vi "AVI Video Save.vi"(5 "Frame Size":u32, 6 "Channel":T1, 7 "AVI mode":T6, 8 "error in (no error)":errorcluster, 9 "AVI cluster":T2, 10 "PMT is ON?":bool, 11 "Image Pixels":i16[][](array[numeric])) -> (0 "error out":errorcluster, 2 "New split file has just been initialised":bool)   [LabVIEW 2017]
uses:
  Typedefs/AVI implementation enum.ctl
  Typedefs/AVI Refs cluster.ctl
  <vilib>/vision/Avi.llb/IMAQ AVI2 Refnum.ctl
  <vilib>/vision/Image Controls.llb/IMAQ Image.ctl
  <vilib>/vision/Avi1.llb/AviRefnum.ctl
  Typedefs/Channel Selector.ctl
  Globals/gl_Binary time series files globals.vi
panel:
  in  "file (use dialog) 2":path=path "X:/Microscope data/2015-July-31/Binary data 2.bin"
  in  "file (use dialog)":path=path "X:/Microscope data/2015-July-31/Binary data 1.bin"
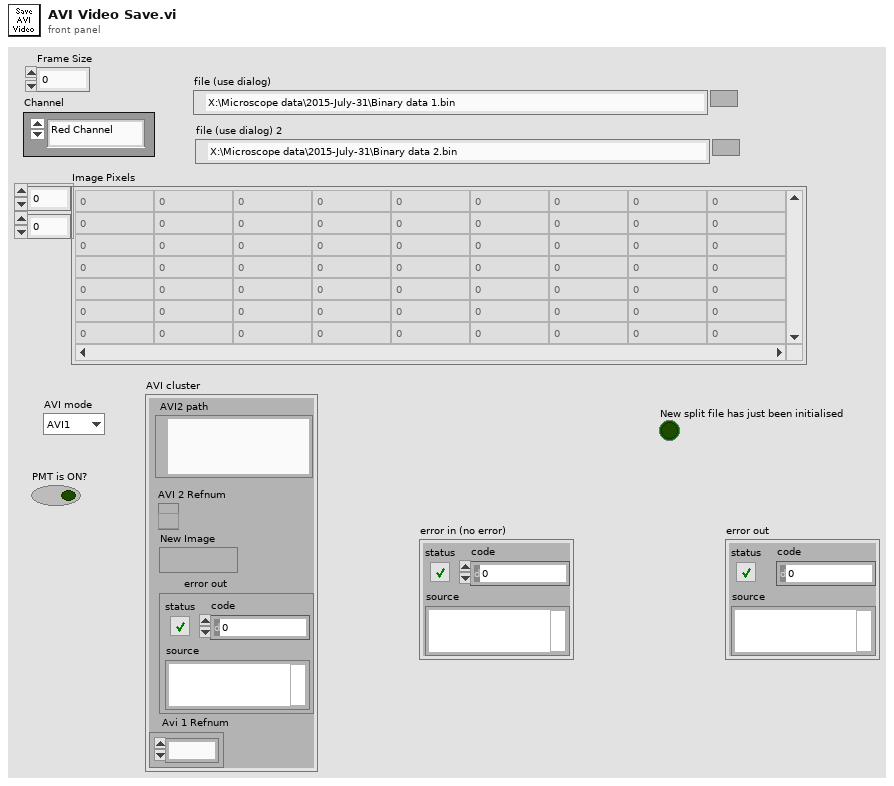
[diagram p1: front panel]
types:
  T1 = typedef "Channel Selector.ctl" = enum16{"Red Channel", "Green Channel", "Blended"}
  T2 = typedef "AVI Refs cluster.ctl" = cluster{"AVI2 path":path, "AVI 2 Refnum":T3, "New Image":T4, "error out":errorcluster, "Avi 1 Refnum":T5}
  T3 = typedef "IMAQ AVI2 Refnum.ctl" = refnum<k20>
  T4 = typedef "IMAQ Image.ctl" = refnum<image>
  T5 = typedef "AviRefnum.ctl" = refnum<k1>
  T6 = typedef "AVI implementation enum.ctl" = enum16{"AVI1", "AVI2"}
  T7 = enum16{"open", "replace", "create", "open or create", "replace or create", "replace or create with confirmation"}
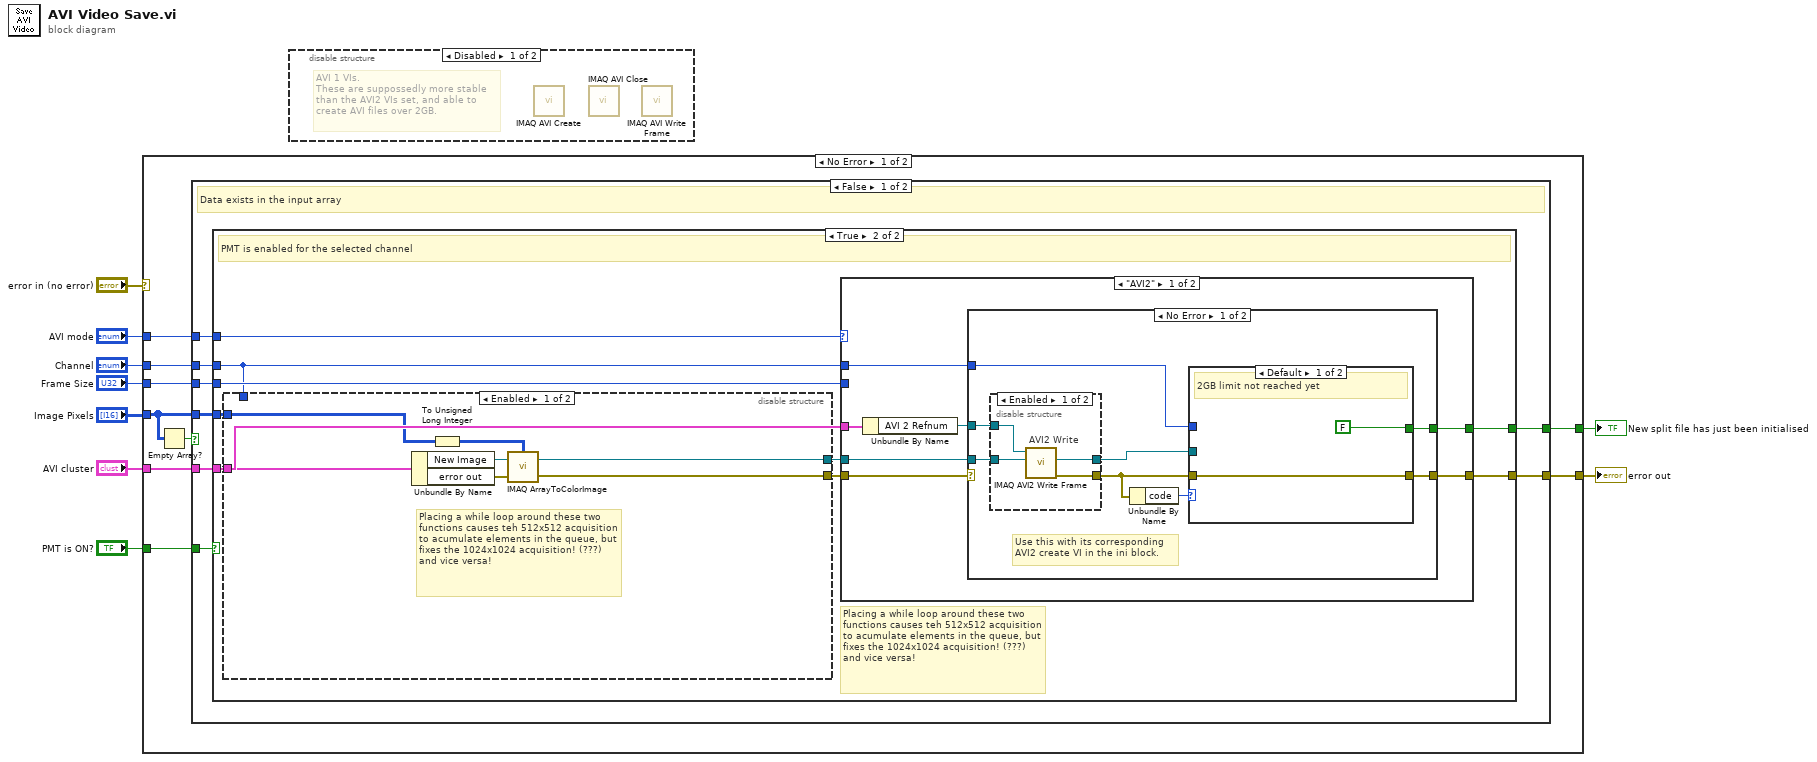
[diagram p0: block diagram]
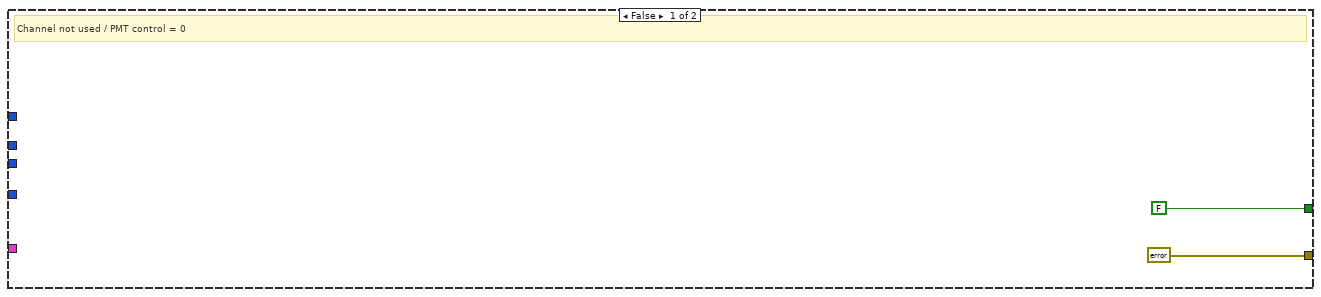
[diagram p3: hidden frame]
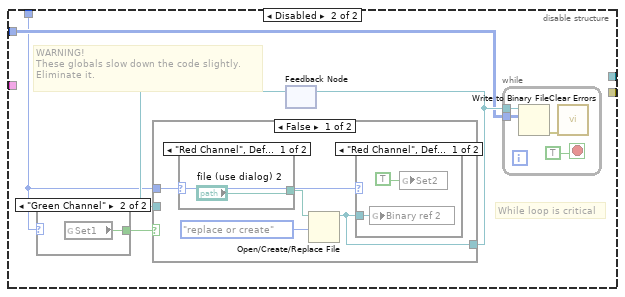
[diagram p4: hidden frame]
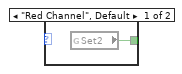
[diagram p5: hidden frame]
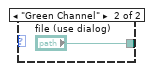
[diagram p6: hidden frame]
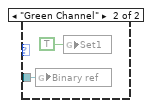
[diagram p7: hidden frame]
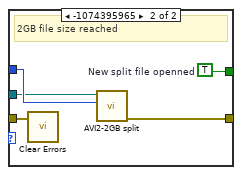
[diagram p10: hidden frame]
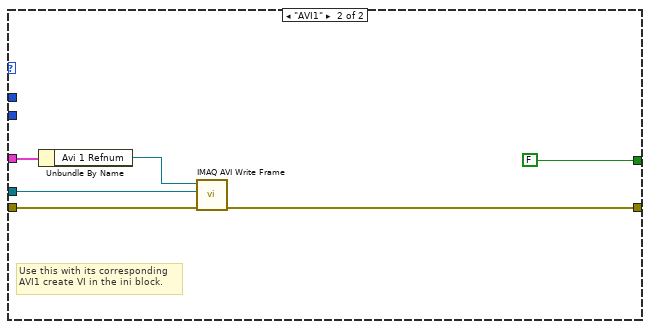
[diagram p12: hidden frame]
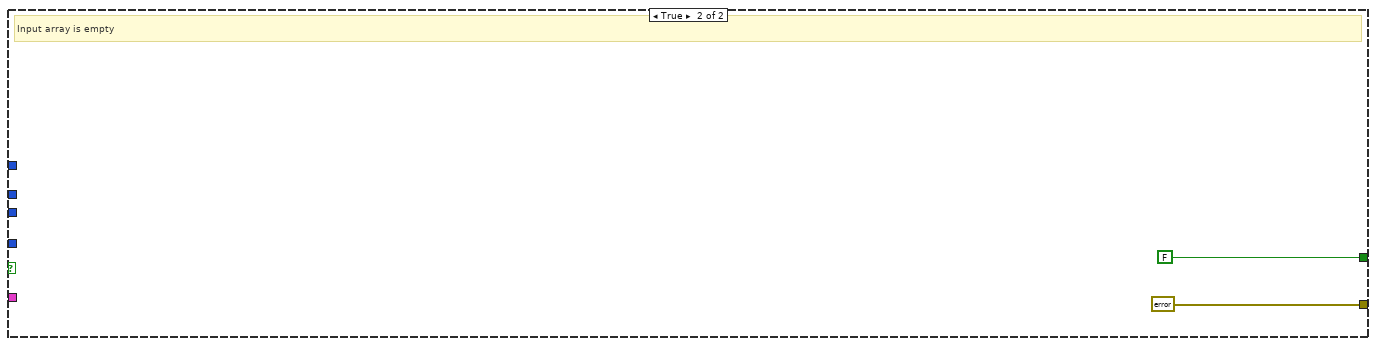
[diagram p13: hidden frame]
diagram:
  n1 = case shown="No Error" "error in (no error)" {
    tunnel: [w18 _] -> w7
    tunnel: "Image Pixels" -> [w10 _]
    tunnel: "AVI mode" -> [w17 _]
    tunnel: "AVI cluster" -> [w16 _]
    tunnel: "PMT is ON?" -> [w15 _]
    tunnel: "Channel" -> [w14 _]
    tunnel: [w13 _] -> w2
    tunnel: "Frame Size" -> [w12 _]
    frame No Error {
      n2 = Empty Array?(array=w10) -> (empty?=w11:bool)
      n3 = case shown="False" w11 {
        tunnel: w10 -> [w26 _]
        tunnel: [w25 errorcluster {"status"=FALSE, "code"=0, "source"=""} ("error out")] -> w18
        tunnel: w17 -> [w24 _]
        tunnel: w16 -> [w23 _]
        tunnel: w15 -> [w22 _]
        tunnel: w14 -> [w21 _]
        tunnel: [w20 FALSE] -> w13
        tunnel: w12 -> [w19 _]
        frame False {
          # "Data exists in the input array"
          n4 = case shown="True" w22 {
            tunnel: w26 -> [_ w30]
            tunnel: w23 -> [_ w33]
            tunnel: [errorcluster {"status"=FALSE, "code"=0, "source"=""} ("error out") w35] -> w25
            tunnel: w24 -> [_ w34]
            tunnel: w21 -> [_ w29]
            tunnel: [FALSE w32] -> w20
            tunnel: w19 -> [_ w31]
            frame False {
              # "Channel not used / PMT control = 0"
            }
            frame True {
              # "Placing a while loop around these two functions causes teh 512x512 acquisition to acumulate elements in the queue, but fixes the 1024x1024 acquisition! (???)  and vice versa!"
              # "PMT is enabled for the selected channel"
              n5 = disable-structure shown="Enabled" {
                disable-tunnel: [w44 _] -> w37
                disable-tunnel: [w43 _] -> w36
                disable-tunnel: w33 -> [w40 _]
                disable-tunnel: w30 -> [w38 w47]
                disable-tunnel: w29 -> [_ w45]
                frame Enabled {
                  # "Placing a while loop around these two functions causes teh 512x512 acquisition to acumulate elements in the queue, but fixes the 1024x1024 acquisition! (???)  and vice versa!"
                  n6 = Unbundle By Name(w40) -> ("New Image"=w42:T4, "error out"=w41:errorcluster)
                  n7 = To Unsigned Long Integer(number=w38) -> (unsigned 32bit integer=w39:u32[][])
                  n8 = call "IMAQ ArrayToColorImage"("Image Pixels (U32)"=w39, "Image"=w42, "error in (no error)"=w41) -> ("Image Out"=w43:T4, "error out"=w44:errorcluster)  [unwired: 1 in, 1 out]
                }
                frame Disabled {
                  # "WARNING!\nThese globals slow down the code slightly.\nEliminate it."
                  # "While loop is critical"
                  n9 = case shown="\"Green Channel\"" w45 {
                    tunnel: [w50 w51] -> w46
                    frame "Red Channel", Default {
                      n10 = global read "gl_Binary time series files globals.vi" "Set2"() -> (w50:bool)
                    }
                    frame "Green Channel" {
                      n11 = global read "gl_Binary time series files globals.vi" "Set1"() -> (w51:bool)
                    }
                  }
                  n12 = feedback #1() -> (w48:refnum<file>)  [unwired: 1 in]
                  n13 = case shown="False" w46 {
                    tunnel: [w58 w66] -> w49
                    tunnel: w48 -> [_ w66]
                    tunnel: w45 -> [w56 _]
                    frame False {
                      n14 = case shown="\"Red Channel\", Default" w56 {
                        tunnel: ["file (use dialog) 2" "file (use dialog)"] -> w59
                        frame "Red Channel", Default {
                        }
                        frame "Green Channel" {
                        }
                      }
                      n15 = Open/Create/Replace File(file path (use dialog)=w59, operation (0:open)=T7."replace or create") -> (refnum out=w58:refnum<file>)  [unwired: 4 in, 2 out]
                      n16 = case shown="\"Red Channel\", Default" w56 {
                        tunnel: w58 -> [w63 w65]
                        frame "Red Channel", Default {
                          n17 = global write "gl_Binary time series files globals.vi" "Binary ref 2"(w63) -> ()
                          n18 = global write "gl_Binary time series files globals.vi" "Set2"(TRUE ("Set1")) -> ()
                        }
                        frame "Green Channel" {
                          n19 = global write "gl_Binary time series files globals.vi" "Binary ref"(w65) -> ()
                          n20 = global write "gl_Binary time series files globals.vi" "Set1"(TRUE ("Set1")) -> ()
                        }
                      }
                    }
                    frame True {
                    }
                  }
                  n21 = feedback-in #1(w49) -> ()
                  n22 = while {
                    tunnel: w49 -> [w55]
                    tunnel: w47 -> [w54]
                    stop <- TRUE stop-if-true
                    n23 = Write to Binary File(file (use dialog)=w55, data=w54) -> (error out=w53:errorcluster)  [unwired: 4 in, 2 out]
                    n24 = call <vilib>:"Clear Errors.vi"("error in (no error)"=w53) -> ()  [unwired: 5 in, 2 out]
                  }
                }
              }
              n25 = case shown="\"AVI2\"" w34 {
                tunnel: w37 -> [w73 w100]
                tunnel: w36 -> [w72 w99]
                tunnel: [w70 w98] -> w35
                tunnel: w33 -> [w71 w96]
                tunnel: w29 -> [w69 _]
                tunnel: [w68 FALSE] -> w32
                tunnel: w31 -> [_ _]
                frame "AVI2" {
                  n26 = Unbundle By Name(w71) -> ("AVI 2 Refnum"=w67:T3)
                  n27 = case shown="No Error" w73 {
                    selector: w73 -> [_ w94]
                    tunnel: w72 -> [w77 _]
                    tunnel: [w81 w94] -> w70
                    tunnel: w69 -> [w80 _]
                    tunnel: w67 -> [w79 _]
                    tunnel: [w75 _] -> w68
                    frame No Error {
                      # "Use this with its corresponding\nAVI2 create VI in the ini block."
                      n28 = disable-structure shown="Enabled" {
                        disable-tunnel: w79 -> [w85 _]
                        disable-tunnel: [w84 _] -> w78
                        disable-tunnel: w77 -> [w83 w86]
                        disable-tunnel: [w82 w86] -> w74
                        frame Enabled {
                          # "AVI2 Write"
                          n29 = call "IMAQ AVI2 Write Frame"("Image"=w83, "AVI Refnum"=w85) -> ("error out"=w84:errorcluster, "Image Out (duplicate)"=w82:T4)  [unwired: 7 in, 1 out]
                        }
                        frame Disabled {
                        }
                      }
                      n30 = Unbundle By Name(w78) -> ("code"=w76:i32)
                      n31 = case shown="Default" w76 {
                        tunnel: [w88 w91] -> w81
                        tunnel: w80 -> [_ w93]
                        tunnel: w78 -> [w88 w92]
                        tunnel: [FALSE w89] -> w75
                        tunnel: w74 -> [_ w90]
                        frame Default {
                          # "2GB limit not reached yet"
                        }
                        frame -1074395965 {
                          w89 = TRUE  # New split file openned
                          # "2GB file size reached"
                          n32 = call <vilib>:"Clear Errors.vi"("error in (no error)"=w92) -> ()  [unwired: 5 in, 2 out]
                          n33 = call "AVI2-2GB split.vi"("Channel"=w93, "Timelapse frame that couldn't be written"=w90) -> ("error out"=w91:errorcluster)  [unwired: 9 in]
                        }
                      }
                    }
                    frame Error {
                    }
                  }
                }
                frame "AVI1" {
                  # "Use this with its corresponding\nAVI1 create VI in the ini block."
                  n34 = Unbundle By Name(w96) -> ("Avi 1 Refnum"=w97:T5)
                  n35 = call "IMAQ AVI Write Frame"("error in (no error)"=w100, "Image"=w99, "Avi Refnum"=w97) -> ("error out"=w98:errorcluster)  [unwired: 7 in, 1 out]
                }
              }
            }
          }
        }
        frame True {
          # "Input array is empty"
        }
      }
    }
    frame Error {
    }
  }
  "error out" <- w7
  "New split file has just been initialised" <- w2
  n36 = disable-structure shown="Disabled" {
    frame Disabled {
      # "AVI 1 VIs.\nThese are suppossedly more stable\nthan the AVI2 VIs set, and able to\ncreate AVI files over 2GB."
      n37 = call "IMAQ AVI Create"() -> ()  [unwired: 10 in, 2 out]
      n38 = call "IMAQ AVI Close"() -> ()  [unwired: 11 in, 1 out]
      n39 = call "IMAQ AVI Write Frame"() -> ()  [unwired: 10 in, 2 out]
    }
    frame Enabled {
    }
  }
